vi "Format Reentrancy String.vi"(9 "Reentrancy Type":T1(ring), 11 "Reentrant?":bool) -> (2 "Reentrancy String":string)   [LabVIEW 2020, in "VI Properties Editor.lvlib"]
doc: "Formats the reentrancy properties into a string to be displayed."
uses:
  VI Properties Editor.lvlib
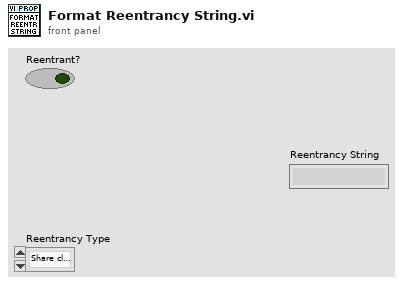
[diagram p1: front panel]
types:
  T1 = enum16{"Share clones between instances", "Preallocate clone for each instance"}
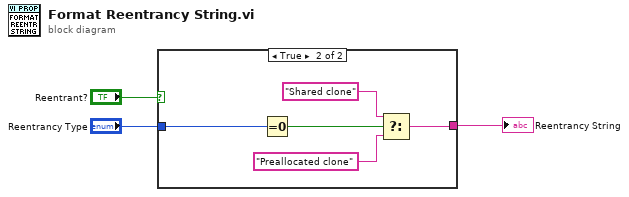
[diagram p0: block diagram]
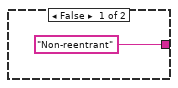
[diagram p2: hidden frame]
diagram:
  n1 = case shown="True" "Reentrant?" {
    tunnel: "Reentrancy Type" -> [_ w9]
    tunnel: ["Non-reentrant" w5] -> w1
    frame False {
    }
    frame True {
      n2 = Equal To 0?(x=w9) -> (x = 0?=w8:bool)
      n3 = Select(t="Shared clone", s=w8, f="Preallocated clone") -> (s? t:f=w5:string)
    }
  }
  "Reentrancy String" <- w1
